vi "Write LogicIO Lookup Table (label -_ LogicIO Obj DVR).vi"(10 "LogicIO Lookup Table (label -> LogicIO Obj DVR)":variant, 11 "VacuumLine in":refnum<class "VacuumLine.lvclass">) -> (3 "VacuumLine out":refnum<class "VacuumLine.lvclass">)   [LabVIEW 2016, in "Hardware.lvlib" / "VacuumLine.lvlib" / "VacuumLine.lvclass"]
uses:
  <userlib>/Common Components/Hardware/Abstract System/VacuumLine/VacuumLine/VacuumLine.lvclass
  <userlib>/Common Components/Hardware/Abstract System/VacuumLine/VacuumLine/VacuumLine.lvclass/VacuumLine.ctl
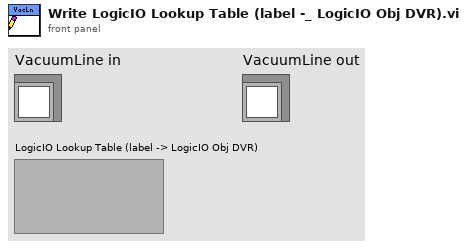
[diagram p1: front panel]
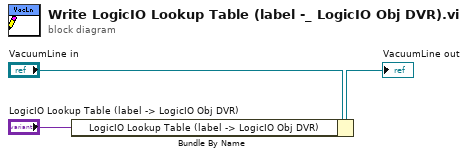
[diagram p0: block diagram]
diagram:
  n1 = Bundle By Name(cluster="VacuumLine in", "LogicIO Lookup Table (label -> LogicIO Obj DVR)"="LogicIO Lookup Table (label -> LogicIO Obj DVR)") -> (→"VacuumLine out":refnum<class "VacuumLine.lvclass">)
